vi "Stock Broker.vi"() -> ()   [LabVIEW 2018]
panel:
  in  "Quit":bool
  in  "Sell Stock":bool
  in  "Buy Stock":bool
  out "Number of Stocks Owned":dbl
  out "Price of Stock/£":dbl format="%#.2g"
  out "Your Money/£":dbl format="%#.2f"
  out "Stock Performance":dbl(graph)
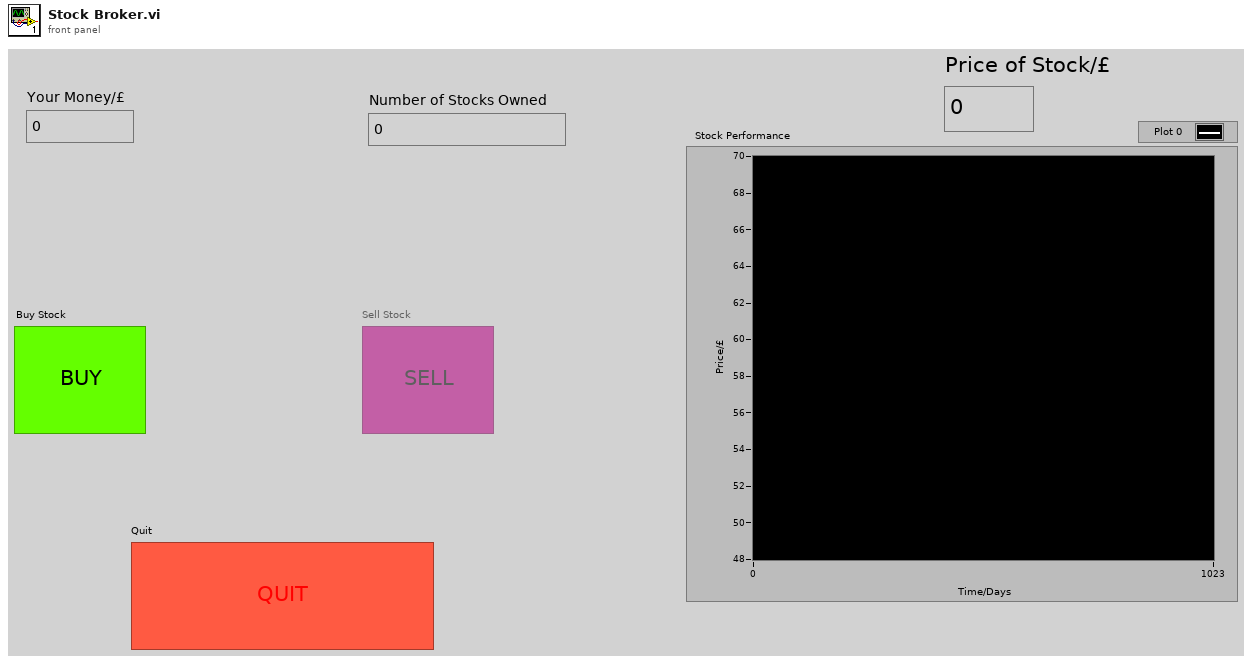
[diagram p1: front panel]
types:
  T1 = enum8{"Enabled", "Disabled", "Disabled and Grayed Out"}
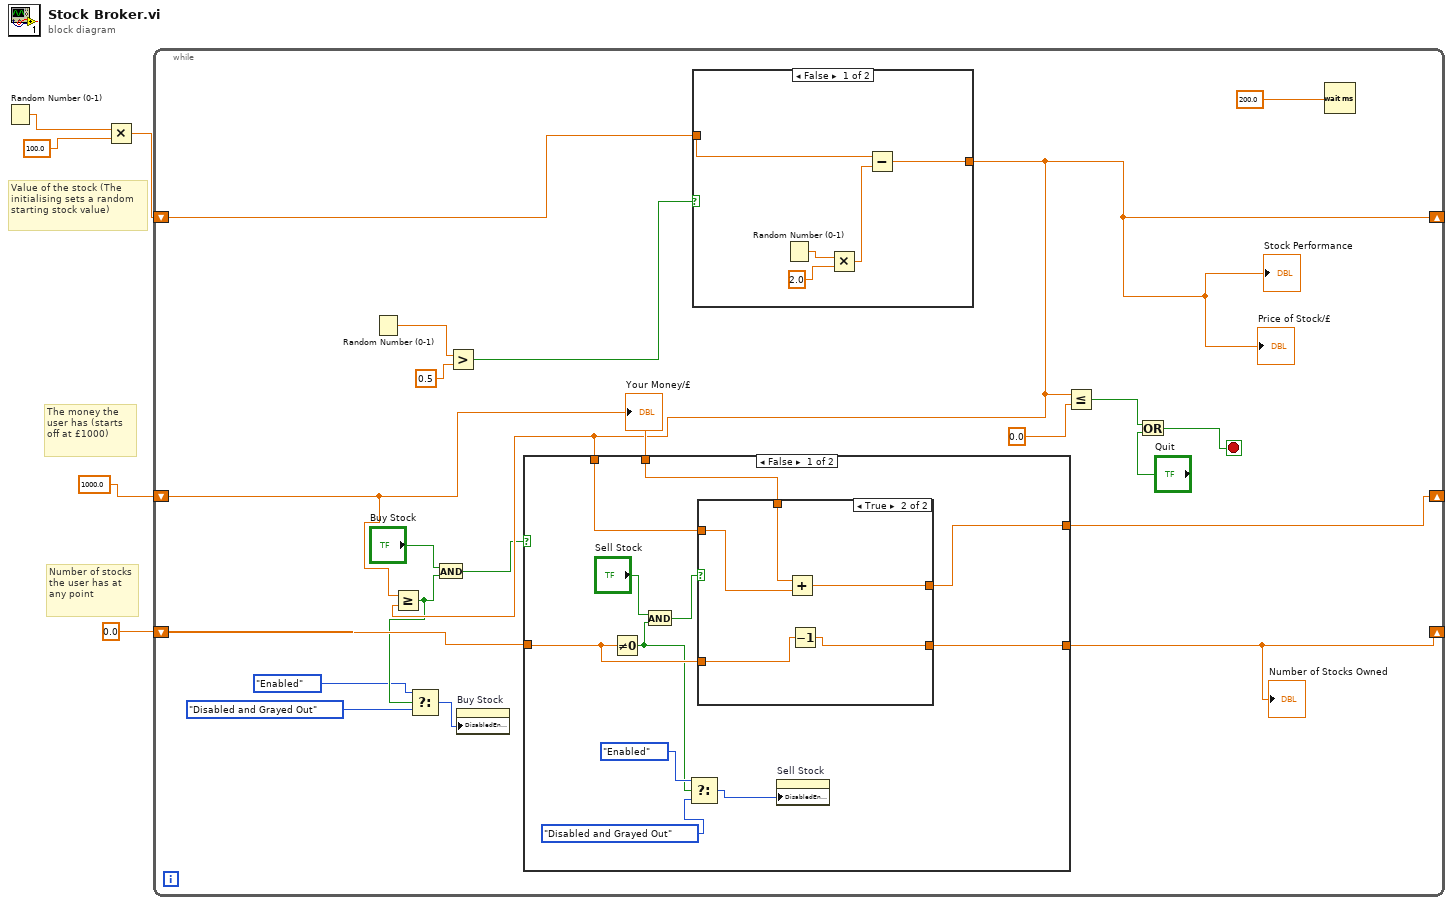
[diagram p0: block diagram]
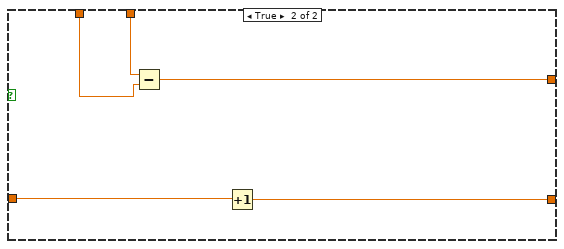
[diagram p3: hidden frame]
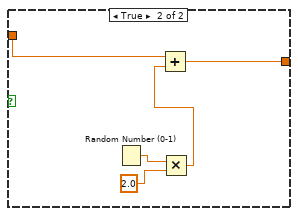
[diagram p4: hidden frame]
diagram:
  # "Value of the stock (The initialising sets a random starting stock value)"
  # "The money the user has (starts off at £1000)"
  # "Number of stocks the user has at any point"
  n1 = Random Number (0-1)() -> (number: 0 to 1=w5:dbl)
  n2 = Multiply(x=w5, y=100.0) -> (x*y=w3:dbl)
  n3 = while {
    shift-right: [w11] -> _
    shift-left: w3 -> [w22]
    shift-right: [w16] -> _
    shift-left: 1000.0 -> [w12]
    shift-right: [w14] -> _
    shift-left: 0.0 -> [w15]
    stop <- w17 stop-if-true
    n4 = Random Number (0-1)() -> (number: 0 to 1=w25:dbl)
    n5 = Greater?(x=w25, y=0.5) -> (0:w23:bool)
    n6 = case shown="False" w23 {
      tunnel: w22 -> [w53 w58]
      tunnel: [w49 w54] -> w11
      frame False {
        n7 = Random Number (0-1)() -> (number: 0 to 1=w52:dbl)
        n8 = Multiply(x=w52, y=2.0) -> (x*y=w50:dbl)
        n9 = Subtract(x=w53, y=w50) -> (x-y=w49:dbl)
      }
      frame True {
        n10 = Random Number (0-1)() -> (number: 0 to 1=w57:dbl)
        n11 = Multiply(x=w57, y=2.0) -> (x*y=w55:dbl)
        n12 = Add(x=w58, y=w55) -> (x+y=w54:dbl)
      }
    }
    "Stock Performance" <- w11
    "Price of Stock/£" <- w11
    n13 = Greater Or Equal?(x=w12, y=w11) -> (x >= y?=w8:bool)
    n14 = Select(t=T1."Enabled" ("Disabled"), s=w8, f=T1."Disabled and Grayed Out" ("Disabled")) -> (s? t:f=w9:T1)
    n15 = And(x="Buy Stock", y=w8) -> (x .and. y?=w10:bool)
    n16 = property on="Buy Stock" class="Bool"("DisabledEnum"=w9) -> ()  [unwired: 2 in, 2 out]
    n17 = case shown="False" w10 {
      tunnel: w12 -> [w36 w48]
      tunnel: w11 -> [w35 w47]
      tunnel: [w34 w46] -> w16
      tunnel: w15 -> [w31 w45]
      tunnel: [w30 w44] -> w14
      frame False {
        n18 = Not Equal To 0?(x=w31) -> (x != 0?=w27:bool)
        n19 = And(x="Sell Stock", y=w27) -> (x .and. y?=w32:bool)
        n20 = Select(t=T1."Enabled" ("Disabled"), s=w27, f=T1."Disabled and Grayed Out" ("Disabled")) -> (s? t:f=w26:T1)
        n21 = case shown="True" w32 {
          tunnel: w36 -> [w38 w43]
          tunnel: w35 -> [_ w42]
          tunnel: [w38 w41] -> w34
          tunnel: w31 -> [w37 w40]
          tunnel: [w37 w39] -> w30
          frame False {
          }
          frame True {
            n22 = Add(x=w43, y=w42) -> (x+y=w41:dbl)
            n23 = Decrement(x=w40) -> (x-1=w39:dbl)
          }
        }
        n24 = property on="Sell Stock" class="Bool"("DisabledEnum"=w26) -> ()  [unwired: 2 in, 2 out]
      }
      frame True {
        n25 = Subtract(x=w48, y=w47) -> (x-y=w46:dbl)
        n26 = Increment(x=w45) -> (x+1=w44:dbl)
      }
    }
    "Number of Stocks Owned" <- w14
    n27 = Less Or Equal?(x=w11, y=0.0) -> (x <= y?=w19:bool)
    n28 = Or(x=w19, y="Quit") -> (x .or. y?=w17:bool)
    n29 = Wait (ms)(milliseconds to wait=200.0) -> ()  [unwired: 1 out]
    "Your Money/£" <- w12
  }
